vi "11.while-wave-form-chart.vi"() -> ()   [LabVIEW 2010]
panel:
  in  "stop":bool
  out "Waveform Chart":dbl(graph)
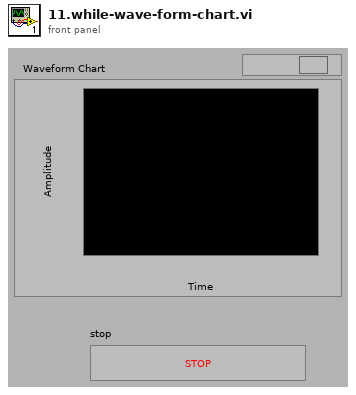
[diagram p1: front panel]
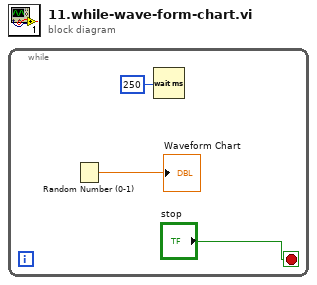
[diagram p0: block diagram]
diagram:
  n1 = while {
    stop <- "stop" stop-if-true
    n2 = Random Number (0-1)() -> (number: 0 to 1=→"Waveform Chart":dbl)
    n3 = Wait (ms)(milliseconds to wait=250) -> ()  [unwired: 1 out]
  }
